vi "Write Rooms List Data.vi"(0 "Rooms List Map":map{string, T1}(c390), 11 "error in (no error)":errorcluster) -> (15 "error out":errorcluster)   [LabVIEW 2023, in "File Data Manager.lvlib" / "File Data Manager.lvclass"]
uses:
  File Data Manager.lvclass
  Central Data Manager/Central Data Manager/Room Details.ctl
  Central Data Manager/Central Data Manager/Room Occupancy Status.ctl
  Central Data Manager/Central Data Manager/Guest Details.ctl
  <vilib>/Utility/file.llb/Write Delimited Spreadsheet (string).vi
  File Data Manager.lvclass/File Data Manager.ctl
  Utilities/Utilities.lvlib
  Central Data Manager/Central Data Manager/Central Data Manager.lvclass
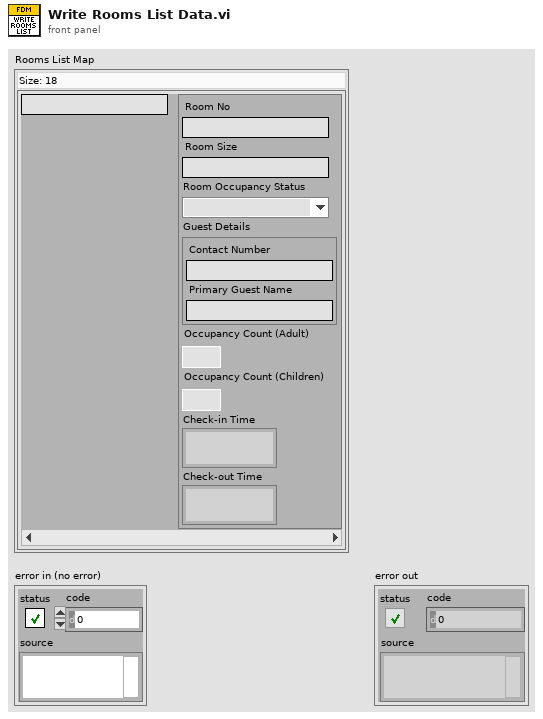
[diagram p1: front panel]
types:
  T1 = typedef "Central Data Manager.lvlib/Central Data Manager.lvclass/Room Details.ctl" = cluster{"Room No":string, "Room Size":string, "Room Occupancy Status":T2, "Guest Details":T3, "Occupancy Count (Adult)":u32, "Occupancy Count (Children)":u32, "Check-in Time":timestamp, "Check-out Time":timestamp}
  T2 = typedef "Central Data Manager.lvlib/Central Data Manager.lvclass/Room Occupancy Status.ctl" = enum16{"Not Occupied", "Occupied", "Under Maintainance", "Not Servicable"}
  T3 = typedef "Central Data Manager.lvlib/Central Data Manager.lvclass/Guest Details.ctl" = cluster{"Contact Number":string, "Primary Guest Name":string}
  T4 = typedef "Hotel Management Tool Model.lvlib/Hotel Management Tool Model.lvclass/Database File Paths.ctl" = cluster{"Food Menu File Path":path, "Guests Histroy File Path":path, "Room Size File Path":path, "Rooms List File Path":path, "Rooms Service Allocation File Path":path, "Staff List File Path":path}
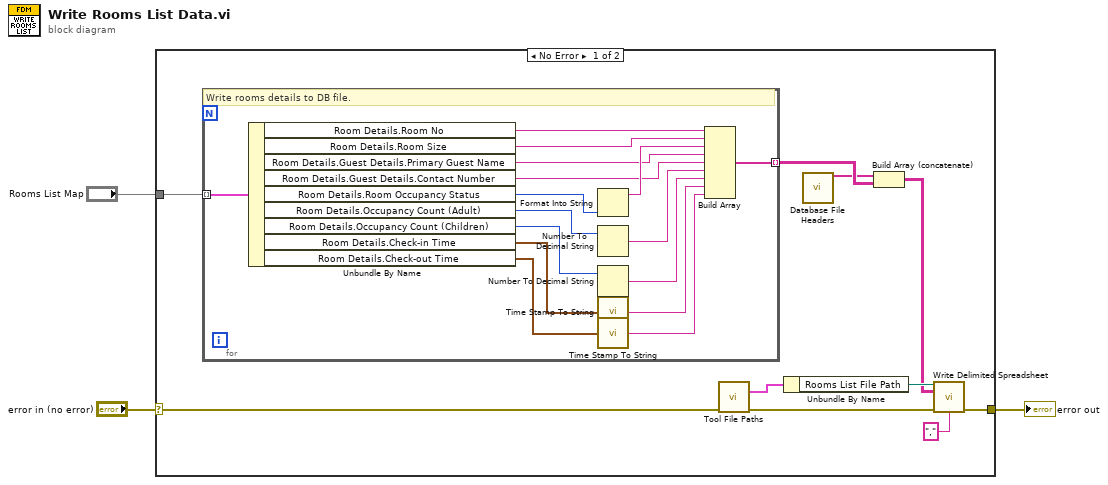
[diagram p0: block diagram]
diagram:
  n1 = case shown="No Error" "error in (no error)" {
    selector: "error in (no error)" -> [w11 w30]
    tunnel: [w7 w30] -> w2
    tunnel: "Rooms List Map" -> [w10 _]
    frame No Error {
      n2 = for {
        tunnel: w10 -> [w29] mode=indexing
        tunnel: [w14] -> w9 mode=indexing
        # "Write rooms details to DB file."
        n3 = Unbundle By Name(w29) -> ("Room Details.Room No"=w28:string, "Room Details.Room Size"=w27:string, "Room Details.Guest Details.Primary Guest Name"=w21:string, "Room Details.Guest Details.Contact Number"=w20:string, "Room Details.Room Occupancy Status"=w15:T2, "Room Details.Occupancy Count (Adult)"=w24:u32, "Room Details.Occupancy Count (Children)"=w23:u32, "Room Details.Check-in Time"=w26:timestamp, "Room Details.Check-out Time"=w25:timestamp)
        n4 = Format Into String(w15) -> (resulting string=w22:string)  [unwired: 3 in, 1 out]
        n5 = Number To Decimal String(number=w24) -> (decimal integer string=w19:string)  [unwired: 1 in]
        n6 = Number To Decimal String(number=w23) -> (decimal integer string=w18:string)  [unwired: 1 in]
        n7 = call "Time Stamp To String.vi"("Time Stamp"=w26) -> ("Output string"=w17:string)
        n8 = call "Time Stamp To String.vi"("Time Stamp"=w25) -> ("Output string"=w16:string)
        n9 = Build Array(w28, w27, w22, w21, w20, w19, w18, w17, w16) -> (w14:string[])
      }
      n10 = call "Tool File Paths.vi"("error in (no error)"=w11) -> ("Database File Paths"=w13:T4, "error out"=w12:errorcluster)  [unwired: 12 in, 1 out]
      n11 = Unbundle By Name(w13) -> ("Rooms List File Path"=w6:path)
      n12 = call "Database File Headers.vi"() -> ("Rooms List Headers"=w8:string[])  [unwired: 13 in, 2 out]
      n13 = Build Array (concatenate)(w8, w9) -> (w4:string[][])
      n14 = call-poly <vilib>:"Write Delimited Spreadsheet.vi"("file path (dialog if empty)"=w6, "2D data"=w4, "error in (no error)"=w12, "delimiter (\\t)"="," ("delimiter (\\t)")) -> ("error out"=w7:errorcluster)  [unwired: 10 in, 1 out]
    }
    frame Error {
    }
  }
  "error out" <- w2
